vi "Autonomous.vi"   [LabVIEW 2017]
doc: "This VI starts when autonomous period begins, and will automatically be terminated when it ends. You can carry out timed or sensor driven operations directly to I/O or to subsystems without needing to return to the caller."
uses:
  <vilib>/Rock Robotics/WPI/Utilities/WPI_GetSetVariantRefNum.vi
  <vilib>/Rock Robotics/Network Tables/NT Read String.vi
types:
  T1 = typedef "WPI_JoystickDevRef.ctl" = cluster{"Device":T2}
  T2 = typedef "WPI_JoystickDeviceEnum.ctl" = enum16{"USB 0", "USB 1", "USB 2", "USB 3", "USB 4", "USB 5"}
  T3 = typedef "Command Status Info.ctl" = cluster{"Name":string, "Status":T4, "notifier out":T5}
  T4 = typedef "Completion Status.ctl" = enum16{"Successful", "Aborted", "Incomplete"}
  T5 = typedef "Completion Notifier.ctl" = refnum<notifier>
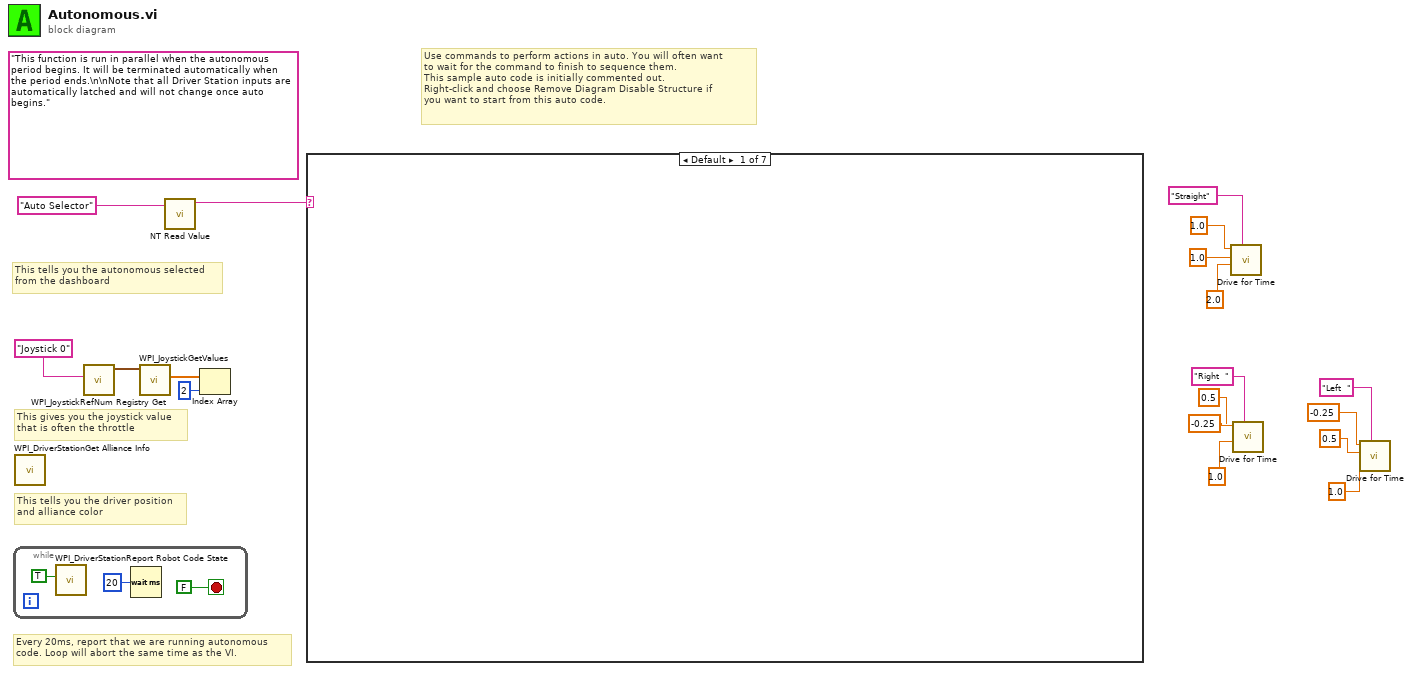
[diagram p0: block diagram]
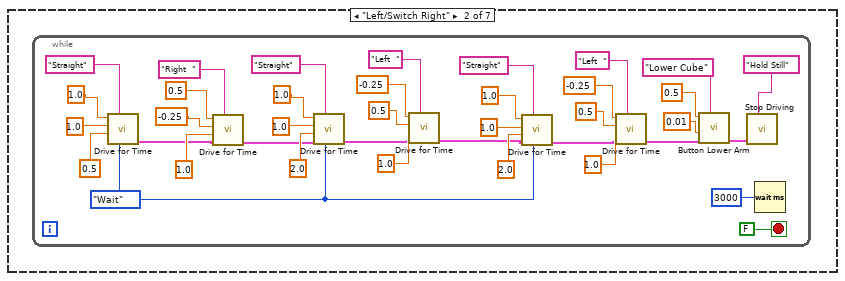
[diagram p2: hidden frame]
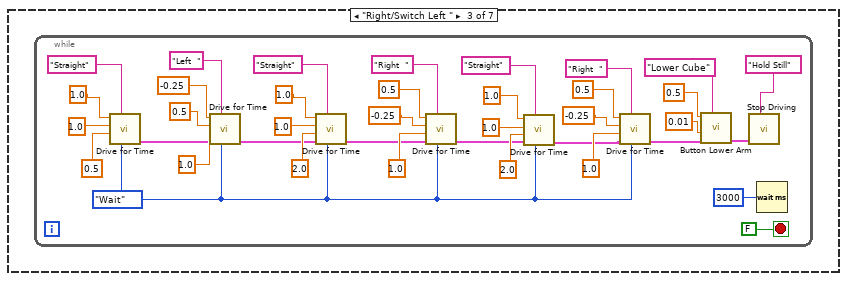
[diagram p3: hidden frame]
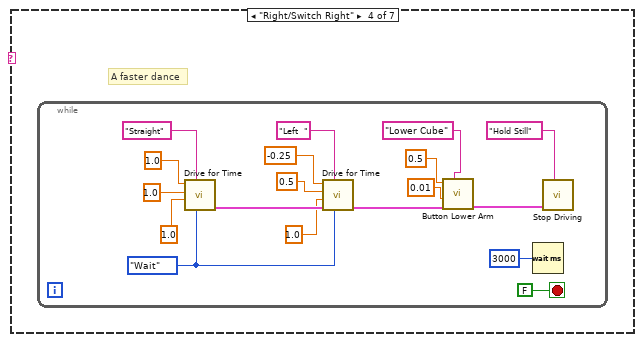
[diagram p4: hidden frame]
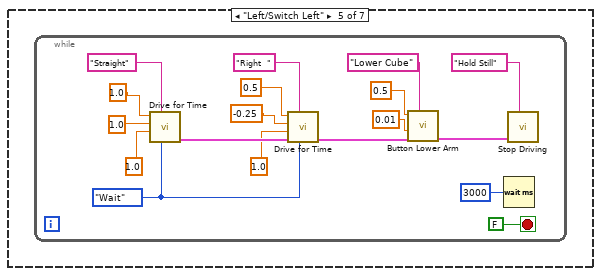
[diagram p5: hidden frame]
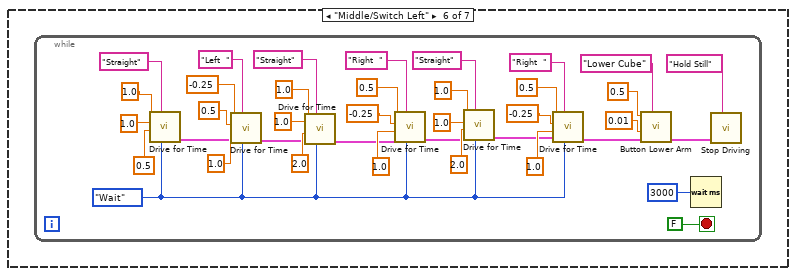
[diagram p6: hidden frame]
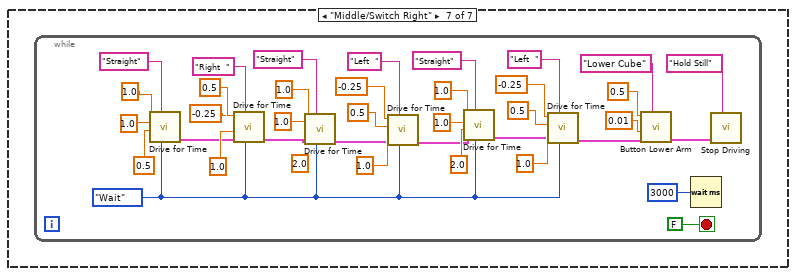
[diagram p7: hidden frame]
diagram:
  (unwired) "This function is run in parallel when the autonomous period begins. It will be terminated automatically when the period ends.\n\nNote that all Driver Station inputs are automatically latched and will not change once auto begins."
  # "Use commands to perform actions in auto. You will often want\nto wait for the command to finish to sequence them.\nThis sample auto code is initially commented out. \nRight-click and choose Remove Diagram Disable Structure if\nyou want to start from this auto code."
  # "This tells you the autonomous selected\nfrom the dashboard"
  # "Every 20ms, report that we are running autonomous\ncode. Loop will abort the same time as the VI."
  # "This gives you the joystick value\nthat is often the throttle"
  # "This tells you the driver position\nand alliance color"
  n1 = while {
    stop <- FALSE stop-if-true
    n2 = call <vilib>:"WPI_DriverStationReport Robot Code State.vi"("Autonomous"=TRUE) -> ()  [unwired: 10 in, 1 out]
    n3 = Wait (ms)(milliseconds to wait=u32 20) -> ()  [unwired: 1 out]
  }
  n4 = call <vilib>:"WPI_DriverStationGet Alliance Info.vi"() -> ()  [unwired: 12 out]
  n5 = call <vilib>:"WPI_JoystickRefNum Registry Get.vi"("refnum name"="Joystick 0") -> ("JoystickDevRef"=w17:T1)  [unwired: 1 in, 9 out]
  n6 = call <vilib>:"WPI_JoystickGetValues.vi"("JoystickDevRef"=w17) -> ("Axes"=w16:dbl[])  [unwired: 6 in, 4 out]
  n7 = call-poly <vilib>:"NT Read Value.vi"("Name"="Auto Selector") -> ("String"=w13:string)  [unwired: 9 in, 1 out]
  n8 = Index Array(array=w16, index=2) -> ()  [unwired: 1 out]
  n9 = case shown="Default" w13 {
    frame Default {
    }
    frame "Left/Switch Right" {
      n10 = while {
        stop <- FALSE stop-if-true
        w40 = enum16{"Start", "Wait"}."Wait" ("Synchronication")
        n11 = call "Drive for Time.vi"("Synchronization"=w40, "Description"="Straight", "Seconds"=0.5 ("Delay (s)"), "Right Speed"=1.0 ("X axis value"), "Left Speed"=1.0 ("X axis value")) -> ("Command Info Out"=w35:T3)  [unwired: 5 in, 1 out]
        n12 = call "Drive for Time.vi"("Description"="Right  ", "Command Info In"=w35, "Seconds"=1.0 ("Delay (s)"), "Right Speed"=-0.25 ("X axis value"), "Left Speed"=0.5 ("X axis value")) -> ("Command Info Out"=w34:T3)  [unwired: 5 in, 1 out]
        n13 = call "Drive for Time.vi"("Synchronization"=w40, "Description"="Straight", "Command Info In"=w34, "Seconds"=2.0 ("Delay (s)"), "Right Speed"=1.0 ("X axis value"), "Left Speed"=1.0 ("X axis value")) -> ("Command Info Out"=w29:T3)  [unwired: 4 in, 1 out]
        n14 = call "Drive for Time.vi"("Description"="Left  ", "Command Info In"=w29, "Seconds"=1.0 ("Delay (s)"), "Right Speed"=0.5 ("X axis value"), "Left Speed"=-0.25 ("X axis value")) -> ("Command Info Out"=w28:T3)  [unwired: 5 in, 1 out]
        n15 = call "Drive for Time.vi"("Synchronization"=w40, "Description"="Straight", "Command Info In"=w28, "Seconds"=2.0 ("Delay (s)"), "Right Speed"=1.0 ("X axis value"), "Left Speed"=1.0 ("X axis value")) -> ("Command Info Out"=w23:T3)  [unwired: 4 in, 1 out]
        n16 = call "Drive for Time.vi"("Description"="Left  ", "Command Info In"=w23, "Seconds"=1.0 ("Delay (s)"), "Right Speed"=0.5 ("X axis value"), "Left Speed"=-0.25 ("X axis value")) -> ("Command Info Out"=w22:T3)  [unwired: 5 in, 1 out]
        n17 = call "Button Lower Arm.vi"("Description"="Lower Cube", "Command Info In"=w22, "Deadband Value"=0.01, "Setpoint"=0.5) -> ("Command Info Out"=w57:T3)  [unwired: 7 in]
        n18 = call "Stop Driving.vi"("Description"="Hold Still", "Command Info In"=w57) -> ()  [unwired: 9 in, 1 out]
        n19 = Wait (ms)(milliseconds to wait=u32 3000 ("millisecond timer value")) -> ()  [unwired: 1 out]
      }
    }
    frame "Right/Switch Left " {
      n20 = while {
        stop <- FALSE stop-if-true
        w60 = enum16{"Start", "Wait"}."Wait" ("Synchronication")
        n21 = call "Drive for Time.vi"("Synchronization"=w60, "Description"="Straight", "Seconds"=0.5 ("Delay (s)"), "Right Speed"=1.0 ("X axis value"), "Left Speed"=1.0 ("X axis value")) -> ("Command Info Out"=w78:T3)  [unwired: 5 in, 1 out]
        n22 = call "Drive for Time.vi"("Synchronization"=w60, "Description"="Left  ", "Command Info In"=w78, "Seconds"=1.0 ("Delay (s)"), "Right Speed"=0.5 ("X axis value"), "Left Speed"=-0.25 ("X axis value")) -> ("Command Info Out"=w73:T3)  [unwired: 4 in, 1 out]
        n23 = call "Drive for Time.vi"("Synchronization"=w60, "Description"="Straight", "Command Info In"=w73, "Seconds"=2.0 ("Delay (s)"), "Right Speed"=1.0 ("X axis value"), "Left Speed"=1.0 ("X axis value")) -> ("Command Info Out"=w72:T3)  [unwired: 4 in, 1 out]
        n24 = call "Drive for Time.vi"("Synchronization"=w60, "Description"="Right  ", "Command Info In"=w72, "Seconds"=1.0 ("Delay (s)"), "Right Speed"=-0.25 ("X axis value"), "Left Speed"=0.5 ("X axis value")) -> ("Command Info Out"=w67:T3)  [unwired: 4 in, 1 out]
        n25 = call "Drive for Time.vi"("Synchronization"=w60, "Description"="Straight", "Command Info In"=w67, "Seconds"=2.0 ("Delay (s)"), "Right Speed"=1.0 ("X axis value"), "Left Speed"=1.0 ("X axis value")) -> ("Command Info Out"=w62:T3)  [unwired: 4 in, 1 out]
        n26 = call "Drive for Time.vi"("Synchronization"=w60, "Description"="Right  ", "Command Info In"=w62, "Seconds"=1.0 ("Delay (s)"), "Right Speed"=-0.25 ("X axis value"), "Left Speed"=0.5 ("X axis value")) -> ("Command Info Out"=w61:T3)  [unwired: 4 in, 1 out]
        n27 = call "Button Lower Arm.vi"("Description"="Lower Cube", "Command Info In"=w61, "Deadband Value"=0.01, "Setpoint"=0.5) -> ("Command Info Out"=w95:T3)  [unwired: 7 in]
        n28 = call "Stop Driving.vi"("Description"="Hold Still", "Command Info In"=w95) -> ()  [unwired: 9 in, 1 out]
        n29 = Wait (ms)(milliseconds to wait=u32 3000 ("millisecond timer value")) -> ()  [unwired: 1 out]
      }
    }
    frame "Right/Switch Right" {
      # "A faster dance"
      n30 = while {
        stop <- FALSE stop-if-true
        w110 = enum16{"Start", "Wait"}."Wait" ("Synchronication")
        n31 = call "Drive for Time.vi"("Synchronization"=w110, "Description"="Straight", "Seconds"=1.0 ("Delay (s)"), "Right Speed"=1.0 ("X axis value"), "Left Speed"=1.0 ("X axis value")) -> ("Command Info Out"=w111:T3)  [unwired: 5 in, 1 out]
        n32 = call "Drive for Time.vi"("Synchronization"=w110, "Description"="Left  ", "Command Info In"=w111, "Seconds"=1.0 ("Delay (s)"), "Right Speed"=0.5 ("X axis value"), "Left Speed"=-0.25 ("X axis value")) -> ("Command Info Out"=w112:T3)  [unwired: 4 in, 1 out]
        n33 = call "Button Lower Arm.vi"("Description"="Lower Cube", "Command Info In"=w112, "Deadband Value"=0.01, "Setpoint"=0.5) -> ("Command Info Out"=w113:T3)  [unwired: 7 in]
        n34 = Wait (ms)(milliseconds to wait=u32 3000 ("millisecond timer value")) -> ()  [unwired: 1 out]
        n35 = call "Stop Driving.vi"("Description"="Hold Still", "Command Info In"=w113) -> ()  [unwired: 9 in, 1 out]
      }
    }
    frame "Left/Switch Left" {
      n36 = while {
        stop <- FALSE stop-if-true
        w121 = enum16{"Start", "Wait"}."Wait" ("Synchronication")
        n37 = call "Drive for Time.vi"("Synchronization"=w121, "Description"="Straight", "Seconds"=1.0 ("Delay (s)"), "Right Speed"=1.0 ("X axis value"), "Left Speed"=1.0 ("X axis value")) -> ("Command Info Out"=w133:T3)  [unwired: 5 in, 1 out]
        n38 = call "Drive for Time.vi"("Synchronization"=w121, "Description"="Right  ", "Command Info In"=w133, "Seconds"=1.0 ("Delay (s)"), "Right Speed"=-0.25 ("X axis value"), "Left Speed"=0.5 ("X axis value")) -> ("Command Info Out"=w118:T3)  [unwired: 4 in, 1 out]
        n39 = call "Button Lower Arm.vi"("Description"="Lower Cube", "Command Info In"=w118, "Deadband Value"=0.01, "Setpoint"=0.5) -> ("Command Info Out"=w116:T3)  [unwired: 7 in]
        n40 = Wait (ms)(milliseconds to wait=u32 3000 ("millisecond timer value")) -> ()  [unwired: 1 out]
        n41 = call "Stop Driving.vi"("Description"="Hold Still", "Command Info In"=w116) -> ()  [unwired: 9 in, 1 out]
      }
    }
    frame "Middle/Switch Left" {
      n42 = while {
        stop <- FALSE stop-if-true
        w134 = enum16{"Start", "Wait"}."Wait" ("Synchronication")
        n43 = call "Drive for Time.vi"("Synchronization"=w134, "Description"="Straight", "Seconds"=0.5 ("Delay (s)"), "Right Speed"=1.0 ("X axis value"), "Left Speed"=1.0 ("X axis value")) -> ("Command Info Out"=w151:T3)  [unwired: 5 in, 1 out]
        n44 = call "Drive for Time.vi"("Synchronization"=w134, "Description"="Left  ", "Command Info In"=w151, "Seconds"=1.0 ("Delay (s)"), "Right Speed"=0.5 ("X axis value"), "Left Speed"=-0.25 ("X axis value")) -> ("Command Info Out"=w146:T3)  [unwired: 4 in, 1 out]
        n45 = call "Drive for Time.vi"("Synchronization"=w134, "Description"="Straight", "Command Info In"=w146, "Seconds"=2.0 ("Delay (s)"), "Right Speed"=1.0 ("X axis value"), "Left Speed"=1.0 ("X axis value")) -> ("Command Info Out"=w141:T3)  [unwired: 4 in, 1 out]
        n46 = call "Drive for Time.vi"("Synchronization"=w134, "Description"="Right  ", "Command Info In"=w141, "Seconds"=1.0 ("Delay (s)"), "Right Speed"=-0.25 ("X axis value"), "Left Speed"=0.5 ("X axis value")) -> ("Command Info Out"=w136:T3)  [unwired: 4 in, 1 out]
        n47 = call "Drive for Time.vi"("Synchronization"=w134, "Description"="Straight", "Command Info In"=w136, "Seconds"=2.0 ("Delay (s)"), "Right Speed"=1.0 ("X axis value"), "Left Speed"=1.0 ("X axis value")) -> ("Command Info Out"=w135:T3)  [unwired: 4 in, 1 out]
        n48 = call "Drive for Time.vi"("Synchronization"=w134, "Description"="Right  ", "Command Info In"=w135, "Seconds"=1.0 ("Delay (s)"), "Right Speed"=-0.25 ("X axis value"), "Left Speed"=0.5 ("X axis value")) -> ("Command Info Out"=w158:T3)  [unwired: 4 in, 1 out]
        n49 = call "Button Lower Arm.vi"("Description"="Lower Cube", "Command Info In"=w158, "Deadband Value"=0.01, "Setpoint"=0.5) -> ("Command Info Out"=w156:T3)  [unwired: 7 in]
        n50 = Wait (ms)(milliseconds to wait=u32 3000 ("millisecond timer value")) -> ()  [unwired: 1 out]
        n51 = call "Stop Driving.vi"("Description"="Hold Still", "Command Info In"=w156) -> ()  [unwired: 9 in, 1 out]
      }
    }
    frame "Middle/Switch Right" {
      n52 = while {
        stop <- FALSE stop-if-true
        (unwired) 2.0 ("Delay (s)")
        w172 = enum16{"Start", "Wait"}."Wait" ("Synchronication")
        n53 = call "Drive for Time.vi"("Synchronization"=w172, "Description"="Straight", "Seconds"=0.5 ("Delay (s)"), "Right Speed"=1.0 ("X axis value"), "Left Speed"=1.0 ("X axis value")) -> ("Command Info Out"=w178:T3)  [unwired: 5 in, 1 out]
        n54 = call "Drive for Time.vi"("Synchronization"=w172, "Description"="Right  ", "Command Info In"=w178, "Seconds"=1.0 ("Delay (s)"), "Right Speed"=-0.25 ("X axis value"), "Left Speed"=0.5 ("X axis value")) -> ("Command Info Out"=w177:T3)  [unwired: 4 in, 1 out]
        n55 = call "Drive for Time.vi"("Synchronization"=w172, "Description"="Straight", "Command Info In"=w177, "Right Speed"=1.0 ("X axis value"), "Left Speed"=1.0 ("X axis value")) -> ("Command Info Out"=w176:T3)  [unwired: 5 in, 1 out]
        n56 = call "Drive for Time.vi"("Synchronization"=w172, "Description"="Left  ", "Command Info In"=w176, "Seconds"=1.0 ("Delay (s)"), "Right Speed"=0.5 ("X axis value"), "Left Speed"=-0.25 ("X axis value")) -> ("Command Info Out"=w175:T3)  [unwired: 4 in, 1 out]
        n57 = call "Drive for Time.vi"("Synchronization"=w172, "Description"="Straight", "Command Info In"=w175, "Seconds"=2.0 ("Delay (s)"), "Right Speed"=1.0 ("X axis value"), "Left Speed"=1.0 ("X axis value")) -> ("Command Info Out"=w174:T3)  [unwired: 4 in, 1 out]
        n58 = call "Drive for Time.vi"("Synchronization"=w172, "Description"="Left  ", "Command Info In"=w174, "Seconds"=1.0 ("Delay (s)"), "Right Speed"=0.5 ("X axis value"), "Left Speed"=-0.25 ("X axis value")) -> ("Command Info Out"=w173:T3)  [unwired: 4 in, 1 out]
        n59 = call "Button Lower Arm.vi"("Description"="Lower Cube", "Command Info In"=w173, "Deadband Value"=0.01, "Setpoint"=0.5) -> ("Command Info Out"=w198:T3)  [unwired: 7 in]
        n60 = Wait (ms)(milliseconds to wait=u32 3000 ("millisecond timer value")) -> ()  [unwired: 1 out]
        n61 = call "Stop Driving.vi"("Description"="Hold Still", "Command Info In"=w198) -> ()  [unwired: 9 in, 1 out]
      }
    }
  }
  n62 = call "Drive for Time.vi"("Description"="Straight", "Seconds"=2.0 ("Delay (s)"), "Right Speed"=1.0 ("X axis value"), "Left Speed"=1.0 ("X axis value")) -> ()  [unwired: 6 in, 2 out]
  n63 = call "Drive for Time.vi"("Description"="Right  ", "Seconds"=1.0 ("Delay (s)"), "Right Speed"=-0.25 ("X axis value"), "Left Speed"=0.5 ("X axis value")) -> ()  [unwired: 6 in, 2 out]
  n64 = call "Drive for Time.vi"("Description"="Left  ", "Seconds"=1.0 ("Delay (s)"), "Right Speed"=0.5 ("X axis value"), "Left Speed"=-0.25 ("X axis value")) -> ()  [unwired: 6 in, 2 out]
